vi "Queue initial values.vi"(8 "error in (no error)":errorcluster, 10 "Run info":T1, 11 "queue":refnum<queue>) -> (0 "error out":errorcluster, 3 "queue out":refnum<queue>)   [LabVIEW 2012]
uses:
  Data.ctl
  Treatment.ctl
  Treatment type.ctl
  <vilib>/Analysis/3filter.llb/Filter Passband Type.ctl
  Run info.ctl
  <vilib>/Analysis/NI_AALBase.lvlib
panel:
  in  "buffer size multiple":dbl=2.0
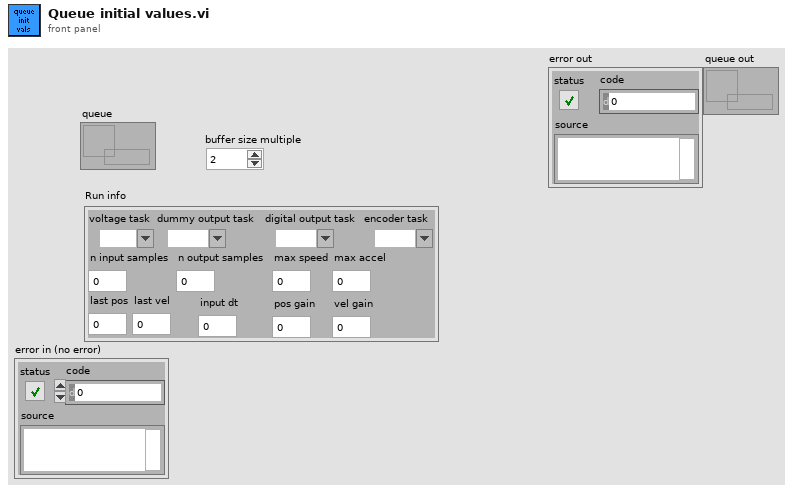
[diagram p1: front panel]
types:
  T1 = typedef "Run info.ctl" = cluster{"voltage task":refnum<k21>, "dummy output task":refnum<k21>, "digital output task":refnum<k21>, "encoder task":refnum<k21>, "n input samples":i32, "n output samples":i32, "max speed":dbl, "max accel":dbl, "last pos":dbl, "last vel":dbl, "pos gain":dbl, "vel gain":dbl, "input dt":dbl}
  T2 = typedef "Data.ctl" = cluster{"Voltage data":dbl[][], "Encoder data":dbl[], "Motor output":dbl[], "Current treatment":T3, "Motor speed":dbl[], "Clipped motor":dbl[], "new treatment":bool}
  T3 = typedef "Treatment.ctl" = cluster{"sample":dbl, "startphase":dbl, "type":T4, "frequency":dbl, "amplitude":dbl, "noise":dbl, "duration":dbl, "kfreq":dbl, "noisehifreq":dbl, "frequency2":dbl, "amplitude2":dbl, "startphase2":dbl, "noise filter type":T5, "noiselofreq":dbl}
  T4 = typedef "Treatment type.ctl" = enum16{"Zero", "Sine", "Frequency sweep", "Two frequency"}
  T5 = typedef "NI_AALBase.lvlib/Filter Passband Type.ctl" = enum32{"Lowpass", "Highpass", "Bandpass", "Bandstop"}
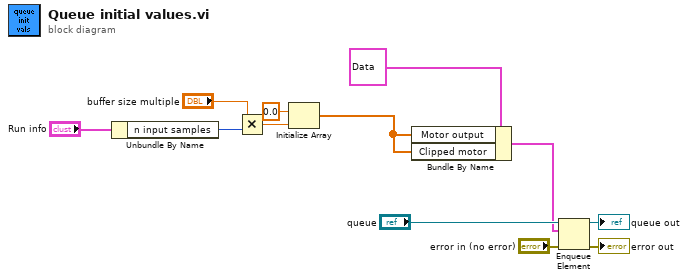
[diagram p0: block diagram]
diagram:
  n1 = Unbundle By Name("Run info") -> ("n input samples"=w9:i32)
  n2 = Multiply(x="buffer size multiple", y=w9) -> (x*y=w7:dbl)
  n3 = Initialize Array(0.0 ("element"), w7) -> (w5:dbl[])
  n4 = Bundle By Name(cluster=T2 {"Voltage data"=[], "Encoder data"=[], "Motor output"=[], "Current treatment"={"sample"=0.0, "startphase"=0.0, "type"=enum."Zero", "frequency"=0.0, "amplitude"=0.0, "noise"=0.0, "duration"=0.0, "kfreq"=0.0, "noisehifreq"=0.0, "frequency2"=0.0, "amplitude2"=0.0, "startphase2"=0.0, "noise filter type"=enum."Lowpass", "noiselofreq"=0.0}, "Motor speed"=[], "Clipped motor"=[], "new treatment"=FALSE} ("element"), "Motor output"=w5, "Clipped motor"=w5) -> (w4:T2)
  n5 = Enqueue Element(queue="queue", element=w4, error in (no error)="error in (no error)") -> (queue out=→"queue out":refnum<queue>, error out=→"error out":errorcluster)  [unwired: 1 in, 1 out]
